vi "Select Automode.vi"(1 "Mode":i32, 2 "Script":string) -> (0 "Output":string)   [LabVIEW 2014]
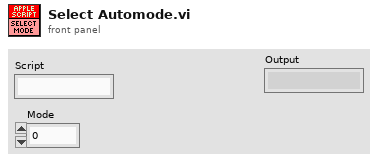
[diagram p1: front panel]
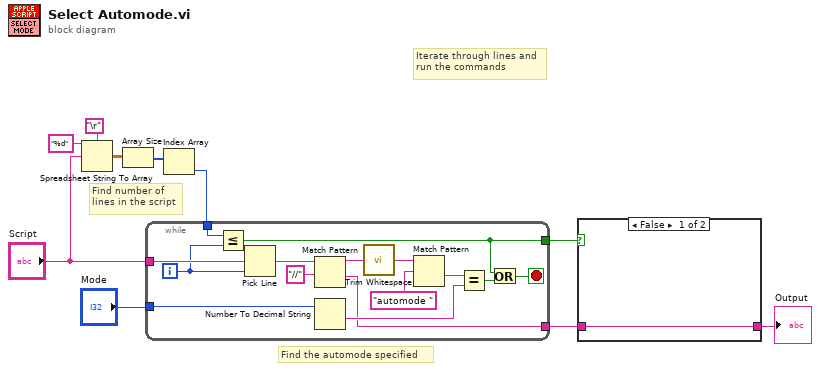
[diagram p0: block diagram]
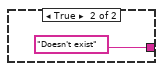
[diagram p2: hidden frame]
diagram:
  # "Find number of \nlines in the script"
  # "Iterate through lines and\nrun the commands"
  # "Find the automode specified"
  n1 = Spreadsheet String To Array(delimiter (Tab)="\r", format string="%d", spreadsheet string="Script") -> (array=w10:dbl[][])  [unwired: 1 in]
  n2 = Array Size(array=w10) -> (size(s)=w7:i32[])
  n3 = Index Array(array=w7) -> (element=w6:i32)  [unwired: 1 in]
  n4 = while {
    tunnel: "Script" -> [w20]
    tunnel: "Mode" -> [w24]
    tunnel: w6 -> [w18]
    tunnel: [w15] -> w3
    tunnel: [w11] -> w2
    i -> [w17]
    stop <- w16 stop-if-true
    n5 = Less Or Equal?(x=w18, y=w17) -> (x <= y?=w15:bool)
    n6 = Pick Line(multi-line string=w20, line index=w17) -> (output string=w12:string)  [unwired: 1 in]
    n7 = Match Pattern(string=w12, regular expression="//" ("search string/char (-)")) -> (before substring=w13:string, after substring=w11:string)  [unwired: 1 in, 2 out]
    n8 = Number To Decimal String(number=w24) -> (decimal integer string=w22:string)  [unwired: 1 in]
    n9 = call <vilib>:"Trim Whitespace.vi"("string"=w13) -> ("trimmed string"=w21:string)  [unwired: 1 in]
    n10 = Match Pattern(string=w21, regular expression="automode ") -> (after substring=w23:string)  [unwired: 1 in, 3 out]
    n11 = Equal?(x=w23, y=w22) -> (x = y?=w19:bool)
    n12 = Or(x=w15, y=w19) -> (x .or. y?=w16:bool)
  }
  n13 = case shown="False" w3 {
    tunnel: w2 -> [w26 _]
    tunnel: [w26 "Doesn't exist" ("output string")] -> w1
    frame False {
    }
    frame True {
    }
  }
  "Output" <- w1
